vi "Read Current Filter.vi"(8 "error in (no error)":errorcluster, 11 "Roda_Filtros in":refnum<class "Roda_Filtros.lvclass">) -> (0 "error out":errorcluster, 2 "Current Filter":u16(ring) items=["Methane", "U", "B", "V", "R", "I", "Clear"], 3 "Roda_Filtros out":refnum<class "Roda_Filtros.lvclass">)   [LabVIEW 2018, in "Roda_Filtros.lvclass"]
uses:
  Roda_Filtros.lvclass
  Roda_Filtros.lvclass/Roda_Filtros.ctl
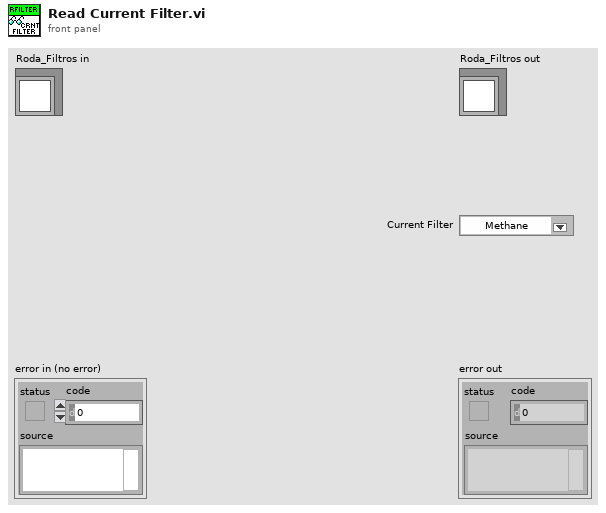
[diagram p1: front panel]
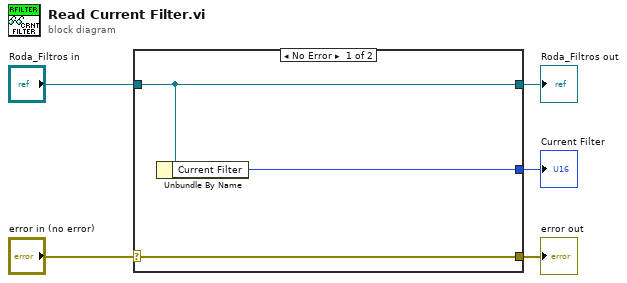
[diagram p0: block diagram]
diagram:
  n1 = case shown="No Error" "error in (no error)" {
    selector: "error in (no error)" -> [w8 w9]
    tunnel: [w8 w9] -> w4
    tunnel: [w7 w10] -> w2
    tunnel: "Roda_Filtros in" -> [w7 w10]
    tunnel: [w6 _] -> w1
    frame No Error {
      n2 = Unbundle By Name(w7) -> ("Current Filter"=w6:u16)
    }
    frame Error {
    }
  }
  "error out" <- w4
  "Roda_Filtros out" <- w2
  "Current Filter" <- w1
